vi "Create Panel.vi"(10 "LVCAM":refnum<class "LVCAM.lvclass">, 11 "ABD Panel in":refnum<class "ABD Panel.lvclass">) -> (0 "error out":errorcluster, 3 "ABD Panel out":refnum<class "ABD Panel.lvclass">)   [LabVIEW 2021, in "ABD Panel.lvclass"]
uses:
  ABD Panel.lvclass
  LVCAM/LVCAM/LVCAM/LVCAM.lvclass
  Main Panel.vi
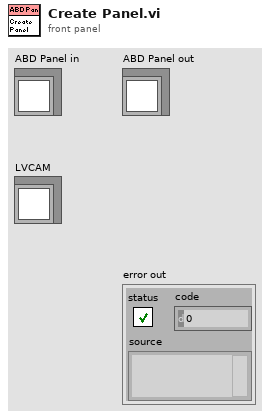
[diagram p1: front panel]
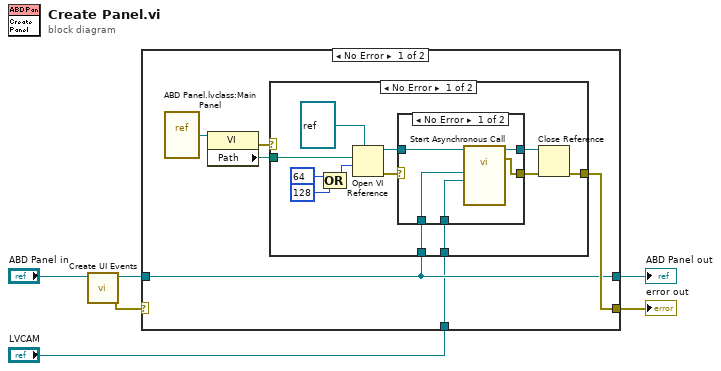
[diagram p0: block diagram]
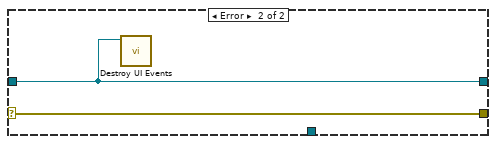
[diagram p4: hidden frame]
diagram:
  n1 = call "Create UI Events.vi"("ABD Panel in"="ABD Panel in") -> ("error out"=w6:errorcluster, "ABD Panel out"=w4:refnum<class "ABD Panel.lvclass">)  [unwired: 9 in]
  n2 = case shown="No Error" w6 {
    selector: w6 -> [_ w34]
    tunnel: [w9 w34] -> w3
    tunnel: w4 -> [w8 w33]
    tunnel: [w8 w33] -> w2
    tunnel: "LVCAM" -> [w7 _]
    frame No Error {
      n3 = vi-ref "ABD Panel.lvclass:Main Panel.vi"() -> (w11:refnum<vi>)
      n4 = property class="VI"(reference=w11) -> (error out=w12:errorcluster, "Path"=w10:path)  [unwired: 1 in, 1 out]
      n5 = case shown="No Error" w12 {
        selector: w12 -> [_ w32]
        tunnel: [w22 w32] -> w9
        tunnel: w10 -> [w18 _]
        tunnel: w8 -> [w14 _]
        tunnel: w7 -> [w13 _]
        frame No Error {
          n6 = Compound Arithmetic op=OR(64 ("options: Multiple Clones,\n  Fire & Forget"), 128 ("options: Multiple Clones,\n  Fire & Forget")) -> (w20:i32)
          n7 = Open VI Reference(type specifier VI Refnum (for type only)=refnum<vi> refnum, vi path=w18, options=w20) -> (vi reference=w16:refnum<vi>, error out=w17:errorcluster)  [unwired: 3 in]
          n8 = case shown="No Error" w17 {
            selector: w17 -> [_ w31]
            tunnel: [w29 w30] -> w24
            tunnel: [w28 w31] -> w23
            tunnel: w16 -> [w27 w30]
            tunnel: w14 -> [w26 _]
            tunnel: w13 -> [w25 _]
            frame No Error {
              n9 = call-by-ref "Start Asynchronous Call"(reference=w27, "LVCAM"=w25, "ABD Panel"=w26) -> (reference out=w29:refnum<vi>, error out=w28:errorcluster)  [unwired: 11 in]
            }
            frame Error {
            }
          }
          n10 = Close Reference(reference=w24, error in (no error)=w23) -> (error out=w22:errorcluster)
        }
        frame Error {
        }
      }
    }
    frame Error {
      n11 = call "Destroy UI Events.vi"("ABD Panel in"=w33) -> ()  [unwired: 11 in]
    }
  }
  "error out" <- w3
  "ABD Panel out" <- w2
